vi "Configure Power Ramp Times.vi"(8 "error in (no error)":errorcluster, 9 "ramp-down time, s":u8, 10 "ramp-up time, s":u8, 11 "HFP Gen in":refnum<class "PL HFP Generator.lvclass">) -> (0 "error out":errorcluster, 3 "HFP Gen out":refnum<class "PL HFP Generator.lvclass">)   [LabVIEW 2015, in "PL HFP Generator.lvclass"]
doc: "Configures power ramp-up and ramp-down times."
uses:
  PL HFP Generator.lvclass
  <vilib>/plasmapper/PL Modbus Client/PL Modbus Client.lvclass
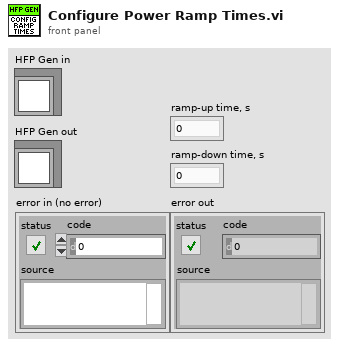
[diagram p1: front panel]
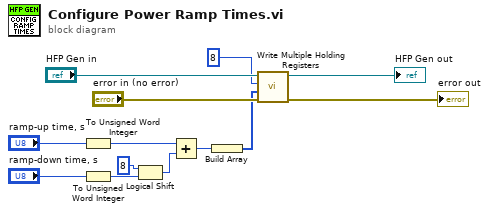
[diagram p0: block diagram]
diagram:
  n1 = To Unsigned Word Integer(number="ramp-up time, s") -> (unsigned 16bit integer=w2:u16)
  n2 = To Unsigned Word Integer(number="ramp-down time, s") -> (unsigned 16bit integer=w5:u16)
  n3 = Logical Shift(y=i16 8, x=w5) -> (x << y=w1:u16)
  n4 = Add(x=w2, y=w1) -> (x+y=w3:u16)
  n5 = Build Array(w3) -> (w8:u16[])
  n6 = call <vilib>:"Write Multiple Holding Registers.vi"("error in (no error)"="error in (no error)", "values"=w8, "address"=u16 8, "MODBUS in"="HFP Gen in") -> ("error out"=→"error out":errorcluster, "MODBUS out"=→"HFP Gen out":refnum<class "PL HFP Generator.lvclass">)  [unwired: 6 in]
